vi "Build Report Path.vi"(8 "error in (no error)":errorcluster, 10 "Start Time":timestamp, 11 "Report Directory":path) -> (0 "error out":errorcluster, 2 "Report Path":path)   [LabVIEW 2020, in "MacroAssert.lvlib"]
doc: "Builds the path to a report file using the provided inputs."
uses:
  MacroAssert.lvlib
  <userlib>/_OpenG.lib/file/file.llb/openg_file.lvlib
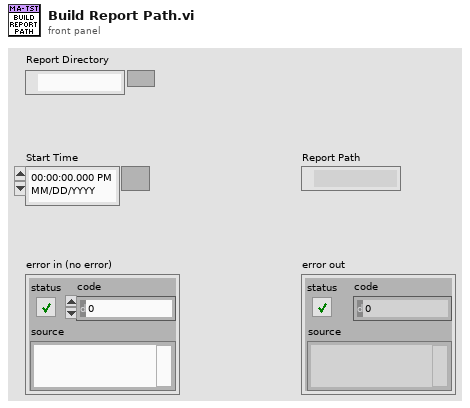
[diagram p1: front panel]
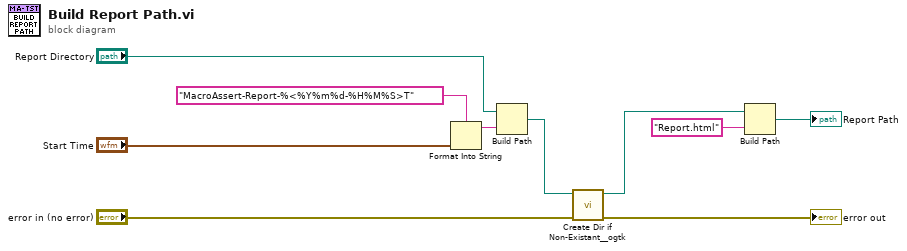
[diagram p0: block diagram]
diagram:
  n1 = Format Into String(format string="MacroAssert-Report-%<%Y%m%d-%H%M%S>T", "Start Time") -> (resulting string=w6:string)  [unwired: 2 in, 1 out]
  n2 = Build Path(base path="Report Directory", name or relative path=w6) -> (appended path=w5:path)
  n3 = call <userlib>:"Create Dir if Non-Existant__ogtk.vi"("error in (no error)"="error in (no error)", "Directory Path"=w5) -> ("error out"=→"error out":errorcluster, "dup Directory Path"=w4:path)  [unwired: 7 in, 1 out]
  n4 = Build Path(base path=w4, name or relative path="Report.html") -> (appended path=→"Report Path":path)
